vi "5051_56_get_inputs.vi"(1 "Address (Main, Sub reqd.)":T1, 2 "Channel Name":string) -> (3 "Comment":string, 4 "All chs.":u16 format="%.0b", 5 "Single Channel":bool, 6 "Single output":dbl format="%.2f")   [LabVIEW 2018]
uses:
  ADAM Client/Sub VIs/ADAM Controls/Address.ctl
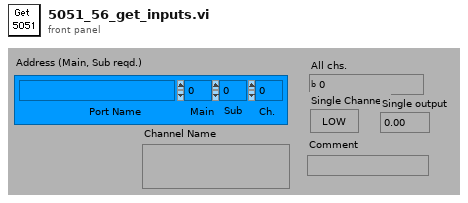
[diagram p1: front panel]
types:
  T1 = typedef "Address.ctl" = cluster{"Main":i32, "Ch.":i32, "Sub":i32, "Port Name":string}
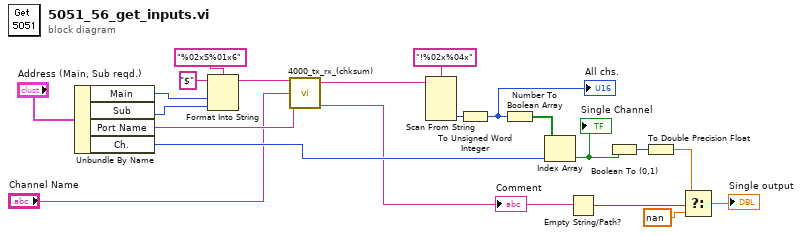
[diagram p0: block diagram]
diagram:
  n1 = Unbundle By Name("Address (Main, Sub reqd.)") -> ("Main"=w20:i32, "Sub"=w21:i32, "Port Name"=w15:string, "Ch."=w13:i32)
  n2 = Format Into String(format string="%02xS%01x6", initial string="$", w20, w21) -> (resulting string=w17:string)  [unwired: 1 in, 1 out]
  n3 = call "4000_tx_rx_(chksum).vi"("Write String"=w17, "Channel Name"="Channel Name", "Port Name"=w15) -> ("Read"=w14:string, "Comment out"=w11:string)  [unwired: 2 in, 1 out]
  "Comment" <- w11
  n4 = Scan From String(format string="!%02x%04x", input string=w14) -> (output 2=w9:u32)  [unwired: 2 in, 6 out]
  n5 = To Unsigned Word Integer(number=w9) -> (unsigned 16bit integer=w12:u16)
  "All chs." <- w12
  n6 = Number To Boolean Array(number=w12) -> (Boolean array=w8:bool[])
  n7 = Index Array(array=w8, index=w13) -> (element=w7:bool)
  "Single Channel" <- w7
  n8 = Empty String/Path?(string/path=w11) -> (empty?=w5:bool)
  n9 = Boolean To (0,1)(Boolean=w7) -> (0, 1=w6:i16)
  n10 = To Double Precision Float(number=w6) -> (double precision float=w3:dbl)
  n11 = Select(t=w3, s=w5, f=nan) -> (s? t:f=→"Single output":dbl)
